vi "GetBatteryVoltage.vi"(11 "packet in":u8[](array[numeric])) -> (3 "battery voltage (V)":dbl)   [LabVIEW 2018]
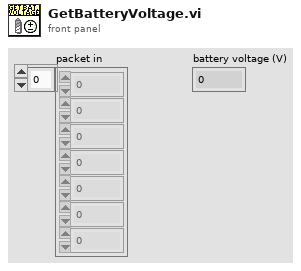
[diagram p1: front panel]
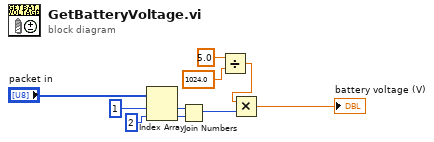
[diagram p0: block diagram]
diagram:
  n1 = Index Array(array="packet in", index #1=1 ("index"), index #2=2 ("index")) -> (element #1=w4:u8, element #2=w5:u8)
  n2 = Join Numbers(hi=w4, lo=w5) -> ((hi.lo)=w9:u16)
  n3 = Divide(x=5.0 ("index"), y=1024.0 ("index")) -> (x/y=w8:dbl)
  n4 = Multiply(x=w8, y=w9) -> (x*y=→"battery voltage (V)":dbl)
